vi "Cull and Group Peg.vi"(6 "Line Border":cluster{"Top":dbl, "Bottom":dbl}={"Top"=6.0, "Bottom"=1.0}, 7 "Bottom Clip":dbl=3.0, 9 "Score Cutoff":dbl=3.0, 10 "Sorted Data":dbl[][](array[numeric])) -> (0 "Rect":T1, 1 "Line":T1, 2 "Score":dbl, 3 "Center":cluster{"X":dbl, "Y":dbl})   [LabVIEW 2016]
doc: "Examine the particle measurements to find the most likely pair that make up the target. This mostly compares the edges of the bounding boxes. It then returns information about the overall target, notably the rectangle sourrounding the particles, the vertical line that bisects the target, and the center of the top particle."
panel:
  out "Grouping Scores":T2(array[cluster])
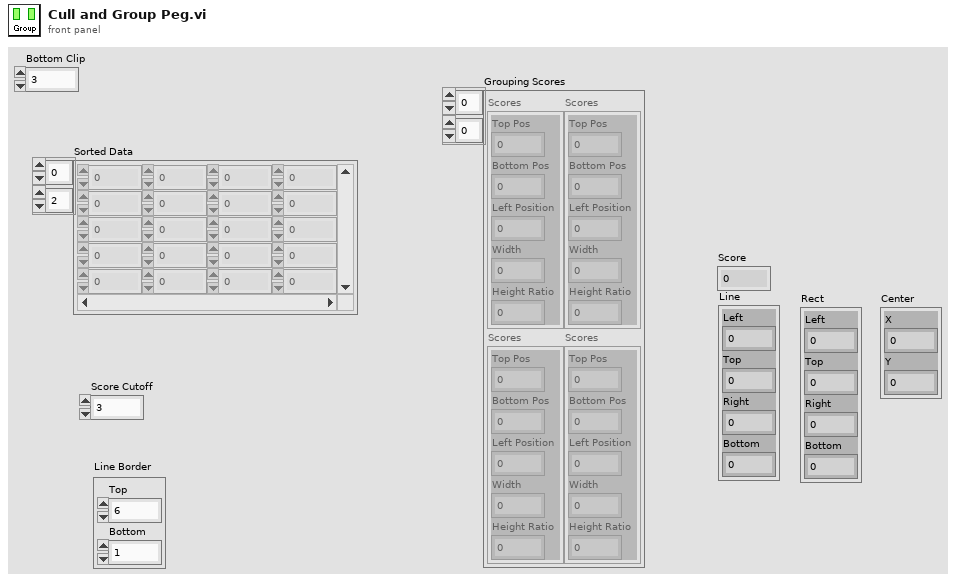
[diagram p1: front panel]
types:
  T1 = cluster{"Left":dbl, "Top":dbl, "Right":dbl, "Bottom":dbl}
  T2 = cluster{"Top Pos":dbl, "Bottom Pos":dbl, "Left Position":dbl, "Width":dbl, "Height Ratio":dbl}[][]
  T3 = cluster{"Top Position":dbl, "Bottom Position":dbl, "Left Gap":dbl, "Width":dbl, "Height Ratio":dbl}
  T4 = cluster{"Left":dbl, "Numeric":dbl, "Right":dbl, "Numeric":dbl}
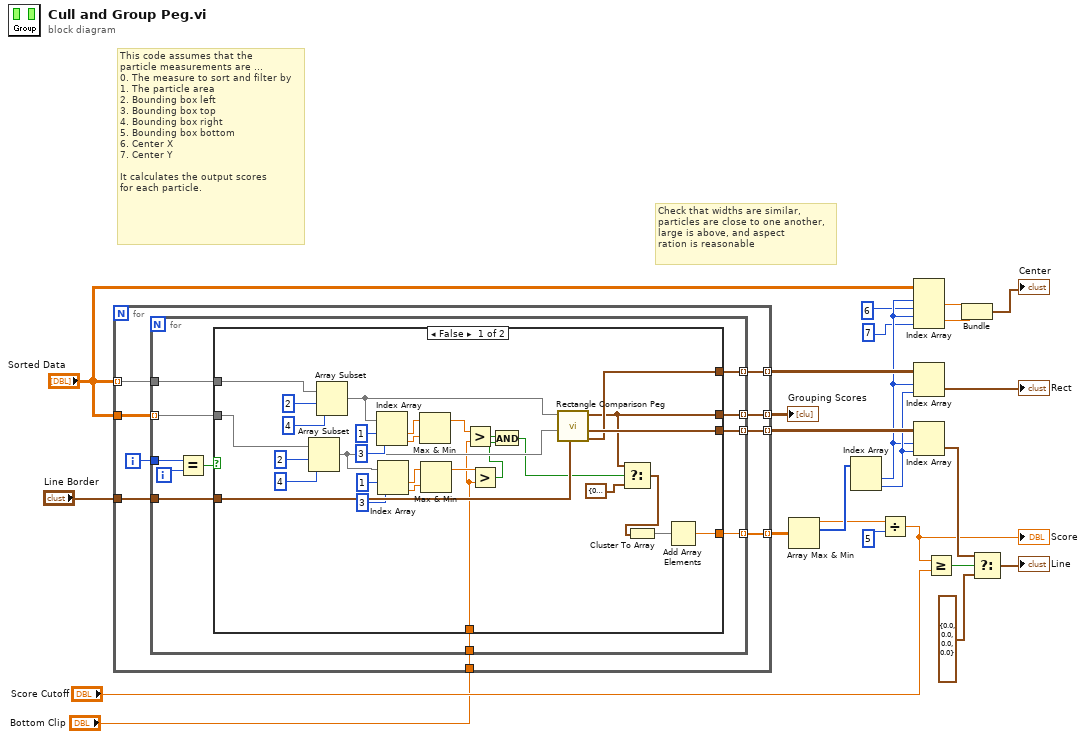
[diagram p0: block diagram]
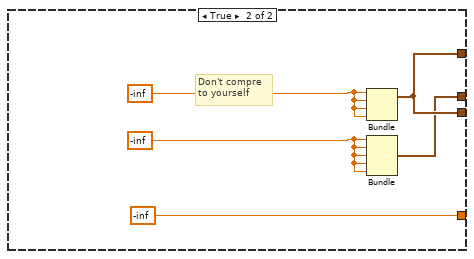
[diagram p2: hidden frame]
diagram:
  # "Check that widths are similar,\nparticles are close to one another,\nlarge is above, and aspect\nration is reasonable"
  # "This code assumes that the\nparticle measurements are ...\n0. The measure to sort and filter by\n1. The particle area\n2. Bounding box left\n3. Bounding box top\n4. Bounding box right\n5. Bounding box bottom\n6. Center X\n7. Center Y\n\nIt calculates the output scores\nfor each particle."
  n1 = for {
    tunnel: "Sorted Data" -> [w33] mode=indexing
    tunnel: "Sorted Data" -> [w32]
    tunnel: [w31] -> w24 mode=indexing
    tunnel: [w29] -> w23 mode=indexing
    tunnel: [w28] -> w20 mode=indexing
    tunnel: [w27] -> w16 mode=indexing
    tunnel: "Line Border" -> [w26]
    tunnel: "Bottom Clip" -> [w25]
    i -> [w30]
    n2 = for {
      tunnel: w33 -> [w44]
      tunnel: w32 -> [w42] mode=indexing
      tunnel: [w41] -> w31 mode=indexing
      tunnel: w30 -> [w40]
      tunnel: [w38] -> w29 mode=indexing
      tunnel: [w37] -> w28 mode=indexing
      tunnel: [w36] -> w27 mode=indexing
      tunnel: w26 -> [w35]
      tunnel: w25 -> [w34]
      i -> [w39]
      n3 = Equal?(x=w40, y=w39) -> (x = y?=w43:bool)
      n4 = case shown="False" w43 {
        tunnel: w44 -> [w72 _]
        tunnel: w42 -> [w69 _]
        tunnel: [w48 w75] -> w41
        tunnel: [w67 -inf] -> w38
        tunnel: [w66 w78] -> w37
        tunnel: [w65 w78] -> w36
        tunnel: w35 -> [w64 _]
        tunnel: w34 -> [w45 _]
        frame False {
          n5 = Array Subset(array=w69, index=2, length=4) -> (w53:dbl[])
          n6 = Array Subset(array=w72, index=2, length=4) -> (w63:dbl[])
          n7 = Index Array(array=w63, index #1=1 ("index"), index #2=3 ("index")) -> (element #1=w60:dbl, element #2=w59:dbl)
          n8 = Index Array(array=w53, index #1=1 ("index"), index #2=3 ("index")) -> (element #1=w56:dbl, element #2=w57:dbl)
          n9 = Max & Min(x=w60, y=w59) -> (max(x,y)=w58:dbl)  [unwired: 1 out]
          n10 = Max & Min(x=w56, y=w57) -> (max(x,y)=w52:dbl)  [unwired: 1 out]
          n11 = Greater?(x=w58, y=w45) -> (0:w51:bool)
          n12 = Greater?(x=w52, y=w45) -> (0:w50:bool)
          n13 = And(x=w51, y=w50) -> (x .and. y?=w47:bool)
          n14 = call "Rectangle Comparison Peg.vi"("Line Border"=w64, "Second"=w53, "First"=w63) -> ("Rect"=w65:T1, "Line"=w66:T1, "Scores"=w48:T3)  [unwired: 6 in]
          n15 = Select(t=w48, s=w47, f=T3 {"Top Position"=0.0, "Bottom Position"=0.0, "Left Gap"=0.0, "Width"=0.0, "Height Ratio"=0.0}) -> (s? t:f=w49:T3)
          n16 = Cluster To Array(cluster=w49) -> (array=w68:dbl[])
          n17 = Add Array Elements(numeric array=w68) -> (sum=w67:dbl)
        }
        frame True {
          w76 = -inf
          w77 = -inf
          # "Don't compre\nto yourself"
          n18 = Bundle(w77, w77, w77, w77) -> (w78:cluster{dbl, dbl, dbl, dbl})  [unwired: 1 in]
          n19 = Bundle(w76, w76, w76, w76, w76) -> (w75:cluster{dbl, dbl, dbl, dbl, dbl})  [unwired: 1 in]
        }
      }
    }
  }
  "Grouping Scores" <- w24
  n20 = Array Max & Min(array=w23) -> (max value=w5:dbl, max index (indices)=w6:i32[])  [unwired: 2 out]
  n21 = Index Array(array=w6) -> (element #1=w12:i32, element #2=w15:i32)  [unwired: 2 in]
  n22 = Divide(x=w5, y=5 ("length")) -> (x/y=w4:dbl)
  "Score" <- w4
  n23 = Index Array(array="Sorted Data", index (row) #1=w12, index (col) #1=6 ("index"), index (row) #2=w12, index (col) #2=7 ("index")) -> (element #1=w10:dbl, element #2=w9:dbl)
  n24 = Index Array(array=w16, index (row)=w12, index (col)=w15) -> (element=→"Rect":T1)
  n25 = Index Array(array=w20, index (row)=w12, index (col)=w15) -> (element=w19:T1)
  n26 = Greater Or Equal?(x=w4, y="Score Cutoff") -> (x >= y?=w22:bool)
  n27 = Bundle("Numeric"=w10, "Numeric"=w9) -> (→"Center":cluster{"Numeric":dbl, "Numeric":dbl})  [unwired: 1 in]
  n28 = Select(t=w19, s=w22, f=cluster{dbl, "Numeric":dbl, dbl, "Numeric":dbl} {0.0, "Numeric"=0.0, 0.0, "Numeric"=0.0}) -> (s? t:f=→"Line":T4)
